vi "Write Multiple Coils.vi"(8 "error in (no error)":errorcluster, 9 "coil values":bool[](array[boolean]), 10 "starting address":u16, 11 "MB CR in":refnum<class "Modbus Master CR API.lvclass">) -> (0 "error out":errorcluster, 3 "MB CR out":refnum<class "Modbus Master CR API.lvclass">)   [LabVIEW 2021, in "Modbus Master CR API.lvclass"]
doc: "Writes values to contiguous coils."
uses:
  Modbus Master CR API.lvclass
  D:/my_projects/projects/Algorithms/Labview/21/Modbus_v121c/API/Modbus API.lvclass
  Modbus API.lvclass/Modbus API.ctl
  Network Protocol/MB/Modbus Master CR.lvclass/Modbus Master CR.ctl
  Read Network Protocol.vi
  Network Protocol/MB/Modbus Master CR.lvclass
  Data Model/Device Data Model.lvclass
  Modbus Master CR API.lvclass/Modbus Master CR API.ctl
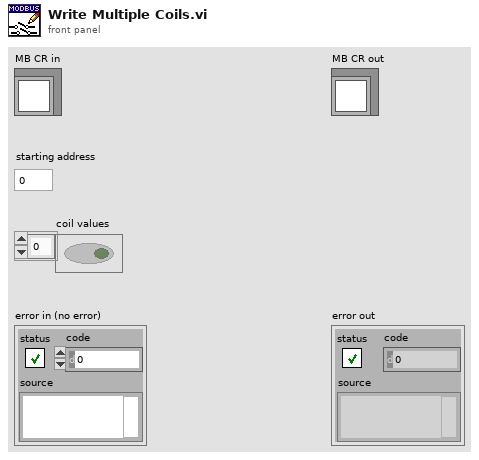
[diagram p1: front panel]
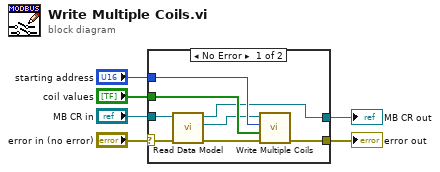
[diagram p0: block diagram]
diagram:
  n1 = case shown="No Error" "error in (no error)" {
    selector: "error in (no error)" -> [w7 w16]
    tunnel: [w12 w16] -> w3
    tunnel: "MB CR in" -> [w8 w15]
    tunnel: "coil values" -> [w14 _]
    tunnel: "starting address" -> [w13 _]
    tunnel: [w9 w15] -> w1
    frame No Error {
      n2 = call "Read Data Model.vi"("error in (no error)"=w7, "MB CR in"=w8) -> ("error out"=w11:errorcluster, "device data model"=w10:refnum<class "Device Data Model.lvclass">, "MB CR out"=w9:refnum<class "Modbus Master CR API.lvclass">)  [unwired: 7 in]
      n3 = call-dynamic "Write Multiple Coils.vi"("error in"=w11, "coils"=w14, "starting address"=w13, "device data model in"=w10) -> ("error out"=w12:errorcluster)  [unwired: 6 in, 1 out]
    }
    frame Error {
    }
  }
  "error out" <- w3
  "MB CR out" <- w1
